vi "AttenRaster.vi"(9 "nRep":i32=4, 10 "n2":i32=10, 11 "n1":i32=11) -> (2 "Atten2 progression":i32[](array[numeric]), 3 "Atten1 progression":i32[](array[numeric]))   [LabVIEW 2012]
panel:
  out "Atten Progression":cluster{i32[], i32[]}[](graph)
  out "Attenarray 2":i32[](array[numeric])
  out "Attenarray 1":i32[](array[numeric])
  out "Index progression":cluster{i32[], i32[]}[](graph)
  out "Atten2 Index":i32[](array[numeric])
  out "Atten1 index":i32[](array[numeric])
  out "i2 now":i32
  out "i1 now":i32
  out "nTotal":i32
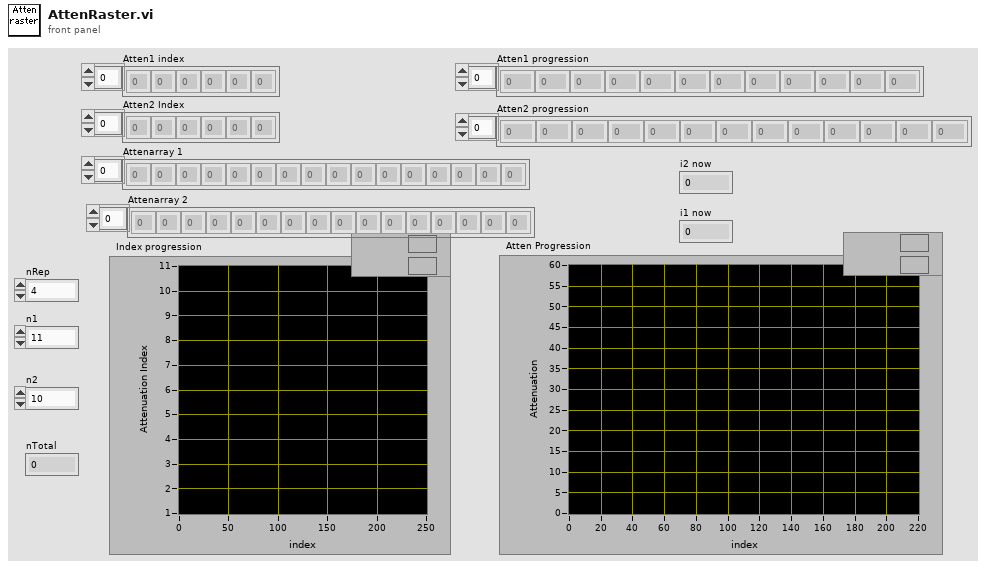
[diagram p1: front panel]
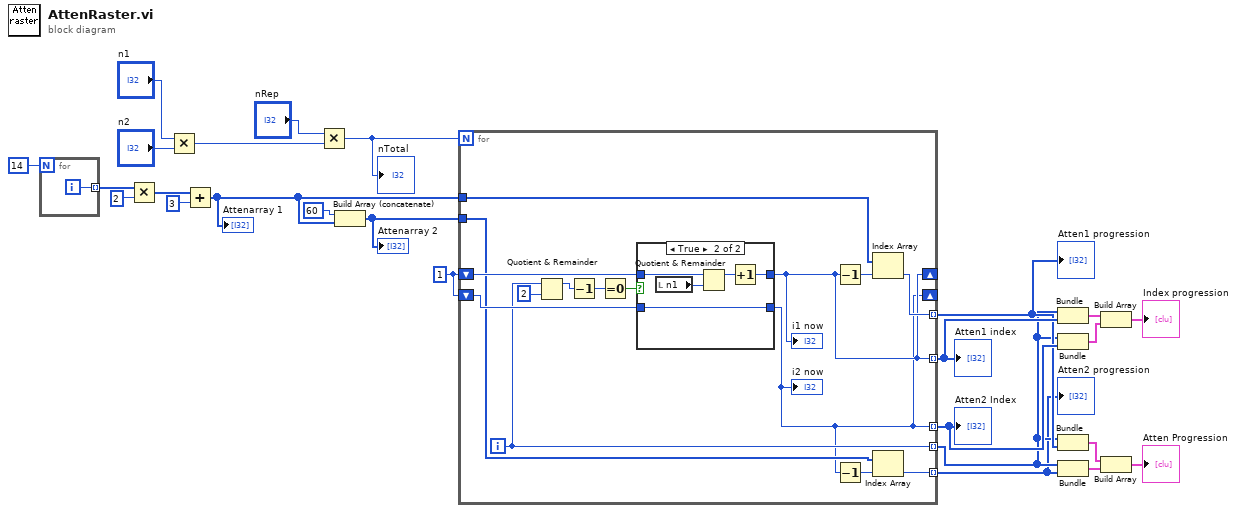
[diagram p0: block diagram]
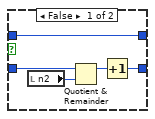
[diagram p2: hidden frame]
diagram:
  w21 = 1
  n1 = for {
    N: 14 -> [_]
    tunnel: [w26] -> w12 mode=indexing
    i -> [w26]
  }
  n2 = Multiply(x=w12, y=2) -> (x*y=w11:i32[])
  n3 = Multiply(x="n1", y="n2") -> (x*y=w23:i32)
  n4 = Add(x=w11, y=3) -> (x+y=w8:i32[])
  "Attenarray 1" <- w8
  n5 = Multiply(x="nRep", y=w23) -> (x*y=w19:i32)
  "nTotal" <- w19
  n6 = Build Array (concatenate)(60 ("y"), w8) -> (w4:i32[])
  "Attenarray 2" <- w4
  n7 = for {
    N: w19 -> [_]
    shift-right: [w30] -> _
    shift-left: w21 -> [w37]
    shift-right: [w28] -> _
    shift-left: w21 -> [w36]
    tunnel: [w30] -> w18 mode=indexing
    tunnel: [w28] -> w20 mode=indexing
    tunnel: [w35] -> w3 mode=indexing
    tunnel: w8 -> [w34]
    tunnel: [w33] -> w7 mode=indexing
    tunnel: w4 -> [w32]
    tunnel: [w31] -> w2 mode=indexing
    i -> [w35]
    n8 = Quotient & Remainder(x=w35, y=2) -> (x-y*floor(x/y)=w41:i32)  [unwired: 1 out]
    n9 = Decrement(x=w41) -> (x-1=w40:i32)
    n10 = Equal To 0?(x=w40) -> (x = 0?=w39:bool)
    n11 = case shown="True" w39 {
      tunnel: w37 -> [w42 w50]
      tunnel: [w42 w48] -> w30
      tunnel: w36 -> [w44 w47]
      tunnel: [w43 w47] -> w28
      frame False {
        n12 = local read "n2"() -> (w46:i32)
        n13 = Quotient & Remainder(x=w44, y=w46) -> (x-y*floor(x/y)=w45:i32)  [unwired: 1 out]
        n14 = Increment(x=w45) -> (x+1=w43:i32)
      }
      frame True {
        n15 = local read "n1"() -> (w51:i32)
        n16 = Quotient & Remainder(x=w50, y=w51) -> (x-y*floor(x/y)=w49:i32)  [unwired: 1 out]
        n17 = Increment(x=w49) -> (x+1=w48:i32)
      }
    }
    "i1 now" <- w30
    "i2 now" <- w28
    n18 = Decrement(x=w30) -> (x-1=w29:i32)
    n19 = Decrement(x=w28) -> (x-1=w27:i32)
    n20 = Index Array(array=w34, index=w29) -> (element=w33:i32)
    n21 = Index Array(array=w32, index=w27) -> (element=w31:i32)
  }
  "Atten1 index" <- w18
  "Atten2 Index" <- w20
  "Atten1 progression" <- w7
  "Atten2 progression" <- w2
  n22 = Bundle(w3, w18) -> (w17:cluster{i32[], i32[]})  [unwired: 1 in]
  n23 = Bundle(w3, w20) -> (w16:cluster{i32[], i32[]})  [unwired: 1 in]
  n24 = Bundle(w3, w7) -> (w5:cluster{i32[], i32[]})  [unwired: 1 in]
  n25 = Bundle(w3, w2) -> (w1:cluster{i32[], i32[]})  [unwired: 1 in]
  n26 = Build Array(w17, w16) -> (→"Index progression":cluster{i32[], i32[]}[])
  n27 = Build Array(w5, w1) -> (→"Atten Progression":cluster{i32[], i32[]}[])
